vi "Example VI.vi"(8 "error in (no error)":errorcluster, 10 "String in":string="Hello World", 11 "Numeric":dbl=1.234) -> (0 "error out":errorcluster, 1 "Greater than 1?":bool, 3 "String out":string)   [LabVIEW 2022 SP3]
doc: "This is a VI Snippet example.\n\nCreated by: Ryan Pacini"
panel:
  out "Indicator":bool
  out "Label.Text":string
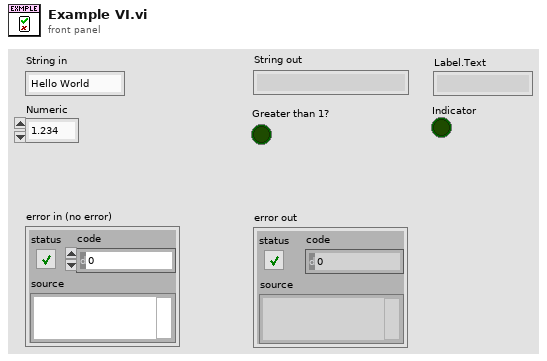
[diagram p1: front panel]
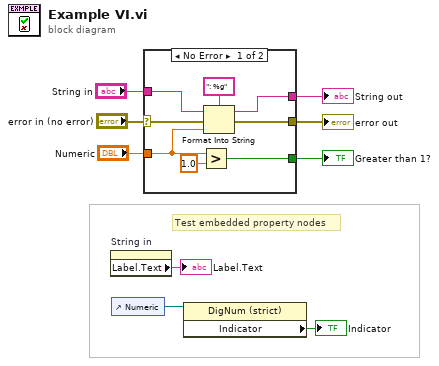
[diagram p0: block diagram]
diagram:
  # "Test embedded property nodes"
  n1 = property on="String in" class="Str"() -> ("Label.Text"=→"Label.Text":string)  [unwired: 2 in, 2 out]
  n2 = control-ref of="Numeric"() -> (w2:refnum<vi>)
  n3 = case shown="No Error" "error in (no error)" {
    selector: "error in (no error)" -> [w17 w18]
    tunnel: "String in" -> [w16 _]
    tunnel: [w14 w18] -> w7
    tunnel: "Numeric" -> [w13 _]
    tunnel: [w11 _] -> w5
    tunnel: [w10 _] -> w4
    frame No Error {
      n4 = Greater?(x=w13, y=1.0) -> (0:w11:bool)
      n5 = Format Into String(format string=": %g", initial string=w16, error in=w17, w13) -> (resulting string=w10:string, error out=w14:errorcluster)
    }
    frame Error {
    }
  }
  "error out" <- w7
  "Greater than 1?" <- w5
  "String out" <- w4
  n6 = property class="DigNum (strict)"(reference=w2) -> ("Indicator"=→"Indicator":bool)  [unwired: 1 in, 2 out]
